vi "node_info.vi"(7 "reference":refnum<vi>, 8 "error in (no error)":errorcluster, 11 "node":string="aaa") -> (0 "error out":errorcluster, 1 "right":string="aaa", 2 "left":string="aaa", 3 "value":i32)   [LabVIEW 2021]
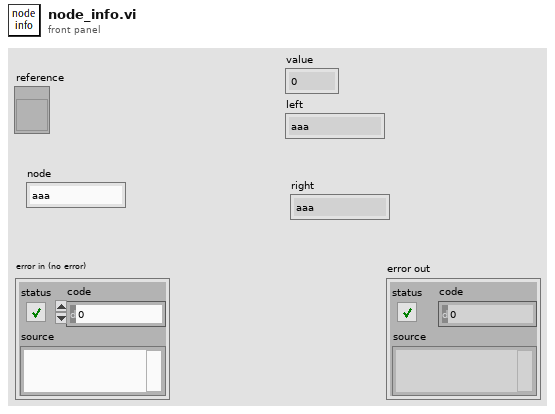
[diagram p1: front panel]
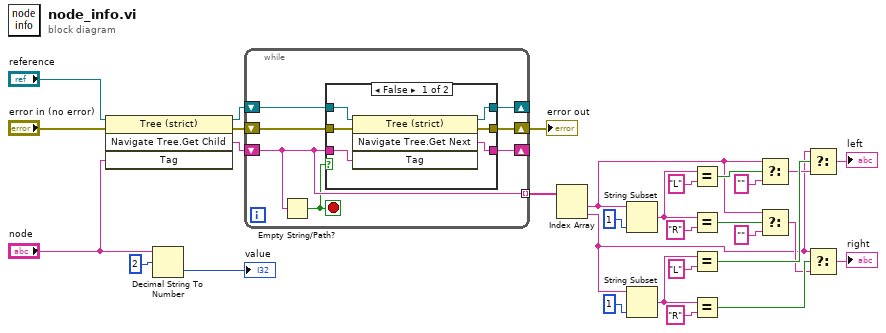
[diagram p0: block diagram]
diagram:
  n1 = invoke on="Invoke Node" class="Tree (strict)" method="Navigate Tree.Get Child"(reference="reference", error in="error in (no error)", "Tag"="node") -> (reference out=w29:refnum<vi>, error out=w28:errorcluster, "Navigate Tree:Get Child"=w27:string)  [unwired: 1 in, 1 out]
  n2 = Decimal String To Number(string="node", offset=2) -> (number=→"value":i32)  [unwired: 1 in, 1 out]
  n3 = while {
    shift-right: [w37] -> _
    shift-left: w27 -> [w32]
    tunnel: [w32] -> w21 mode=indexing
    shift-right: [w35] -> _
    shift-left: w29 -> [w36]
    shift-right: [w33] -> w25
    shift-left: w28 -> [w34]
    stop <- w31 stop-if-true
    n4 = Empty String/Path?(string/path=w32) -> (empty?=w31:bool)
    n5 = case shown="False" w31 {
      tunnel: [w43 w44] -> w37
      tunnel: w36 -> [w39 w46]
      tunnel: [w42 w46] -> w35
      tunnel: w34 -> [w38 w45]
      tunnel: [w41 w45] -> w33
      tunnel: w32 -> [w40 w44]
      frame False {
        n6 = invoke on="Invoke Node" class="Tree (strict)" method="Navigate Tree.Get Next"(reference=w39, error in=w38, "Tag"=w40) -> (reference out=w42:refnum<vi>, error out=w41:errorcluster, "Navigate Tree:Get Next Item"=w43:string)  [unwired: 1 in, 1 out]
      }
      frame True {
      }
    }
  }
  "error out" <- w25
  n7 = Index Array(array=w21) -> (element #1=w14:string, element #2=w1:string)  [unwired: 2 in]
  n8 = String Subset(string=w14, length (rest)=1 ("length (rest)")) -> (substring=w16:string)  [unwired: 1 in]
  n9 = String Subset(string=w1, length (rest)=1 ("length (rest)")) -> (substring=w6:string)  [unwired: 1 in]
  n10 = Equal?(x=w16, y="L") -> (x = y?=w18:bool)
  n11 = Equal?(x=w16, y="R") -> (x = y?=w15:bool)
  n12 = Equal?(x=w6, y="L") -> (x = y?=w10:bool)
  n13 = Equal?(x=w6, y="R") -> (x = y?=w7:bool)
  n14 = Select(t=w14, s=w18, f="") -> (s? t:f=w9:string)
  n15 = Select(t=w14, s=w15, f="") -> (s? t:f=w5:string)
  n16 = Select(t=w1, s=w10, f=w9) -> (s? t:f=→"left":string)
  n17 = Select(t=w1, s=w7, f=w5) -> (s? t:f=→"right":string)
